vi "SanePressures.vi"(8 "Probe Type":u16(ring)=12 items=["5-Hole Probe"=5, "OmniProbe"=12], 11 "ZeroedPressures":dbl[][](array[numeric])) -> (0 "PressureIssues":T1={"PressureErrors"=[], "Plug in titles"=["Good", "AllNegative", "dPTooSmall", "P1smallest", "FailedToReduce", "ExceedMaxCone", "U.LT.0"]}, 2 "XvalsGoodP":i32[](array[numeric]))   [LabVIEW 2016]
doc: "Outputs Xvalues of samples which have acceptable pressures. At least one pressure should be >0, and the difference between the smallest and largest pressures should be greater than the system's noise floor. For the 5HP, P1 should not be the smallest pressure.\nAlso produces diagnostic data for plotting."
uses:
  SanityCluster.ctl
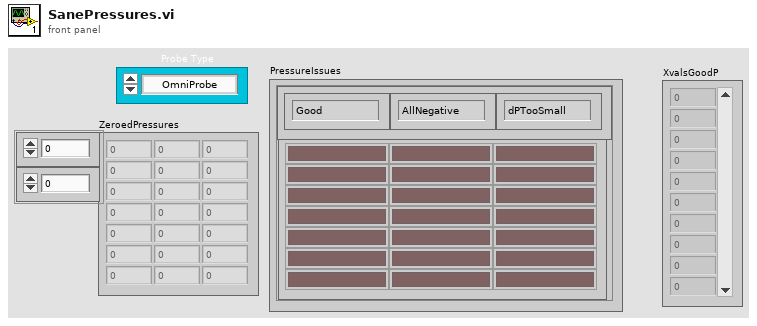
[diagram p1: front panel]
types:
  T1 = typedef "SanityCluster.ctl" = cluster{"PressureErrors":bool[][], "Plug in titles":string[]}
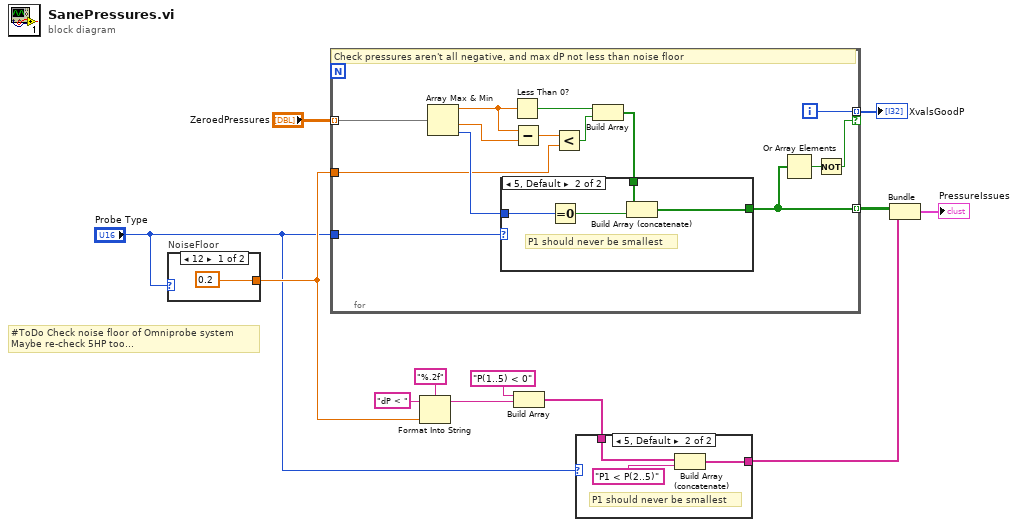
[diagram p0: block diagram]
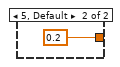
[diagram p2: hidden frame]
diagram:
  # "#ToDo Check noise floor of Omniprobe system\nMaybe re-check 5HP too..."
  n1 = case "NoiseFloor" shown="12" "Probe Type" {
    tunnel: [0.2 ("Minimum dP") 0.2 ("Minimum dP")] -> w3
    frame 12 {
    }
    frame 5, Default {
    }
  }
  n2 = for {
    tunnel: "ZeroedPressures" -> [w19] mode=indexing
    tunnel: [w17] -> w7 mode=indexing
    tunnel: w3 -> [w22]
    tunnel: "Probe Type" -> [w21]
    tunnel: [w18] -> w1 mode=indexing if=w15
    i -> [w18]
    # "Check pressures aren't all negative, and max dP not less than noise floor"
    n3 = Array Max & Min(array=w19) -> (max value=w23:dbl, min value=w24:dbl, min index (indices)=w27:i32)  [unwired: 1 out]
    n4 = Less Than 0?(x=w23) -> (x < 0?=w28:bool)
    n5 = Subtract(x=w23, y=w24) -> (x-y=w25:dbl)
    n6 = Less?(x=w25, y=w22) -> (x < y?=w26:bool)
    n7 = Build Array(w28, w26) -> (w20:bool[])
    n8 = case shown="5, Default" w21 {
      tunnel: w27 -> [_ w33]
      tunnel: w20 -> [w29 w32]
      tunnel: [w29 w30] -> w17
      frame 12 {
        # "P1 could be smallest"
      }
      frame 5, Default {
        # "P1 should never be smallest"
        n9 = Equal To 0?(x=w33) -> (x = 0?=w31:bool)
        n10 = Build Array (concatenate)(w32, w31) -> (w30:bool[])
      }
    }
    n11 = Or Array Elements(Boolean array=w17) -> (logical OR=w16:bool)
    n12 = Not(x=w16) -> (.not. x?=w15:bool)
  }
  "XvalsGoodP" <- w1
  n13 = Format Into String(format string="%.2f", initial string="dP < ", w3) -> (resulting string=w8:string)  [unwired: 1 in, 1 out]
  n14 = Build Array("P(1..5) < 0", w8) -> (w5:string[])
  n15 = case shown="5, Default" "Probe Type" {
    tunnel: w5 -> [w34 w37]
    tunnel: [w34 w36] -> w4
    frame 12 {
      # "Not applicable for Omniprobe"
    }
    frame 5, Default {
      # "P1 should never be smallest"
      n16 = Build Array (concatenate)(w37, "P1 < P(2..5)") -> (w36:string[])
    }
  }
  n17 = Bundle(w7, w4) -> (→"PressureIssues":cluster{bool[][], string[]})  [unwired: 1 in]
